vi "3D Robot Scene.vi"(8 "error in (no error)":errorcluster) -> (0 "error out":errorcluster, 1 "axles":refnum<vi>[](array[refnum]), 2 "robot":refnum<vi>, 3 "scene":refnum<vi>)   [LabVIEW 2015]
doc: "Initializes the 3D drawing of the mecanum robot."
uses:
  <vilib>/picture/3D Picture Control/Object/Create Object (name).vi
  <vilib>/picture/3D Picture Control/NI_3D Picture Control.lvlib
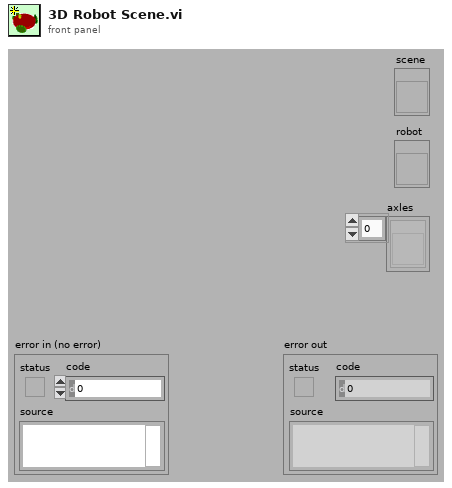
[diagram p1: front panel]
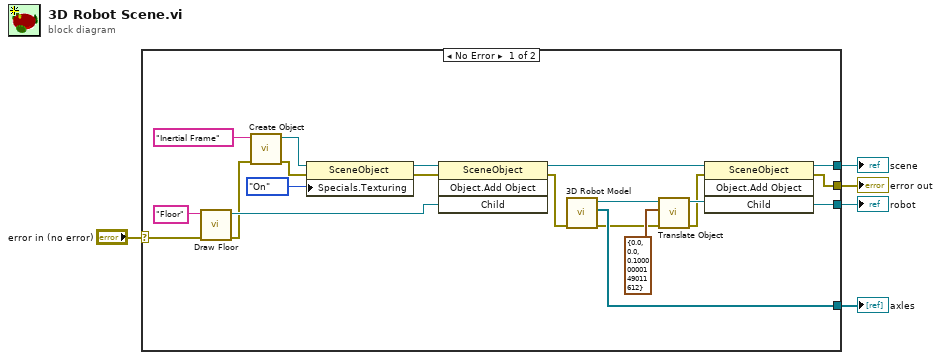
[diagram p0: block diagram]
diagram:
  n1 = case shown="No Error" "error in (no error)" {
    selector: "error in (no error)" -> [w7 w27]
    tunnel: [w26 _] -> w5
    tunnel: [w21 _] -> w4
    tunnel: [w18 _] -> w3
    tunnel: [w6 w27] -> w1
    frame No Error {
      n2 = call "Draw Floor.vi"("error in (no error)"=w7, "name"="Floor" ("Name")) -> ("error out"=w13:errorcluster, "floor object"=w17:refnum<vi>)  [unwired: 8 in]
      n3 = call-poly <vilib>:"Create Object.vi"("error in (no error)"=w13, "Name"="Inertial Frame") -> ("error out"=w12:errorcluster, "Scene:New Object"=w23:refnum<vi>)  [unwired: 8 in]
      n4 = property class="SceneObject"(reference=w23, error in=w12, "Specials.Texturing"=enum16{"Inherit Value", "Off", "On"}."On" ("Specials:Texturing")) -> (reference out=w19:refnum<vi>, error out=w11:errorcluster)
      n5 = invoke class="SceneObject" method="Object.Add Object"(reference=w19, error in=w11, "Child"=w17) -> (reference out=w20:refnum<vi>, error out=w10:errorcluster)  [unwired: 1 in, 2 out]
      n6 = call "3D Robot Model.vi"("error in (no error)"=w10) -> ("error out"=w9:errorcluster, "axles"=w26:refnum<vi>[], "robot frame"=w16:refnum<vi>)  [unwired: 8 in]
      n7 = call <vilib>:"Translate Object.vi"("error in (no error)"=w9, "Translation"=cluster{"X":sgl, "Y":sgl, "Z":sgl} {"X"=0.0, "Y"=0.0, "Z"=0.1}, "Scene.Object In"=w16) -> ("error out"=w8:errorcluster, "Scene.Object Out"=w15:refnum<vi>)  [unwired: 7 in]
      n8 = invoke class="SceneObject" method="Object.Add Object"(reference=w20, error in=w8, "Child"=w15) -> (reference out=w21:refnum<vi>, error out=w6:errorcluster, "Child"=w18:refnum<vi>)  [unwired: 1 in, 1 out]
    }
    frame Error {
    }
  }
  "robot" <- w3
  "axles" <- w5
  "scene" <- w4
  "error out" <- w1
